vi "detect chassis.vi"(8 "error in":errorcluster, 11 "controller in":refnum<class "Controller.lvclass">) -> (0 "error out":errorcluster, 3 "controller out":refnum<class "Controller.lvclass">)   [LabVIEW 2014, in "SMI.lvlib" / "Controller.lvclass"]
uses:
  Controller.lvclass
  SysCfg Device/read system session.vi
  SysCfg Device/write system session.vi
  Chassis/Chassis.lvclass
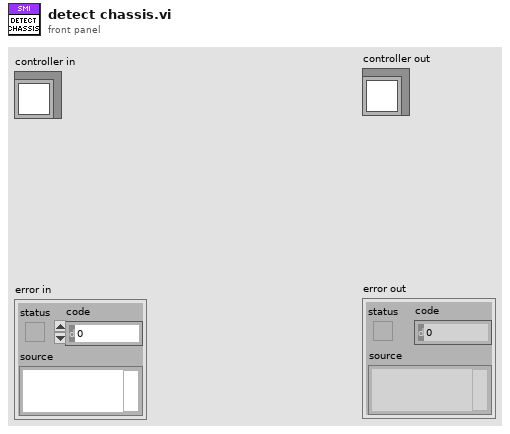
[diagram p1: front panel]
types:
  T1 = typedef "SMI.lvlib/Chassis.lvclass/chassis information.ctl" = cluster{"resource name":string, "vendor name":string, "product name":string, "product ID":u16, "serial number":string, "number of slots":i32, "device class":string}
  T2 = cluster{"local chassis":T1[], "remote chassis":T1[]}
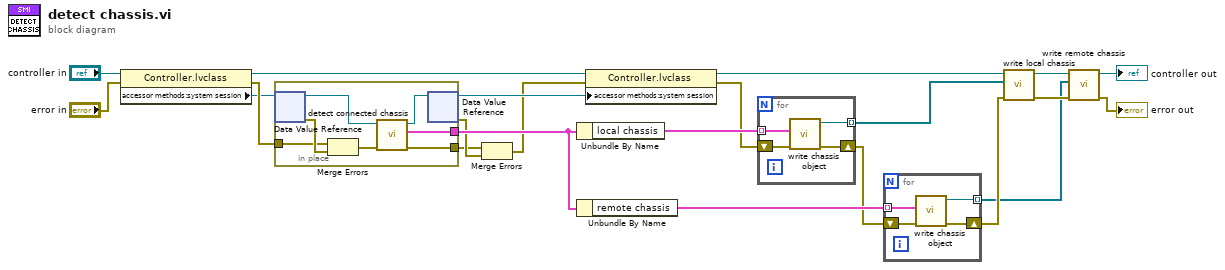
[diagram p0: block diagram]
diagram:
  n1 = property class="Controller.lvclass"(reference="controller in", error in="error in") -> (reference out=w20:refnum<class "Controller.lvclass">, error out=w22:errorcluster, "accessor methods:system session"=w5:refnum<data-value>)
  n2 = in-place {
    in-place-border: w22 -> [w24]
    in-place-border: [w29] -> w1
    in-place-border: [w28] -> w14
    n3 = in-place-dvr #1(w5) -> (w26:refnum<k21>, w25:errorcluster)
    n4 = Merge Errors(w24, w25) -> (w23:errorcluster)
    n5 = call "detect connected chassis.vi"("error in"=w23, "system session in"=w26) -> ("error out"=w29:errorcluster, "chassis"=w28:T2, "system session out"=w27:refnum<k21>)  [unwired: 7 in]
    n6 = in-place-dvr #1(w27) -> (w4:refnum<data-value>, w3:errorcluster)
  }
  n7 = Merge Errors(w1, w3) -> (w2:errorcluster)
  n8 = Unbundle By Name(w14) -> ("local chassis"=w12:T1[])
  n9 = Unbundle By Name(w14) -> ("remote chassis"=w13:T1[])
  n10 = property class="Controller.lvclass"(reference=w20, error in=w2, "accessor methods:system session"=w4) -> (reference out=w6:refnum<class "Controller.lvclass">, error out=w11:errorcluster)
  n11 = for {
    tunnel: w12 -> [w33] mode=indexing
    shift-right: [w31] -> w10
    shift-left: w11 -> [w32]
    tunnel: [w30] -> w9 mode=indexing
    n12 = call "write chassis object.vi"("error in"=w32, "chassis information"=w33) -> ("error out"=w31:errorcluster, "Chassis out"=w30:refnum<class "Chassis.lvclass">)  [unwired: 8 in]
  }
  n13 = for {
    tunnel: w13 -> [w37] mode=indexing
    shift-right: [w35] -> w15
    shift-left: w10 -> [w36]
    tunnel: [w34] -> w8 mode=indexing
    n14 = call "write chassis object.vi"("error in"=w36, "chassis information"=w37) -> ("error out"=w35:errorcluster, "Chassis out"=w34:refnum<class "Chassis.lvclass">)  [unwired: 8 in]
  }
  n15 = call "write local chassis.vi"("error in"=w15, "local chassis"=w9, "controller in"=w6) -> ("error out"=w16:errorcluster, "controller out"=w19:refnum<class "Controller.lvclass">)  [unwired: 7 in]
  n16 = call "write remote chassis.vi"("error in"=w16, "remote chassis"=w8, "controller in"=w19) -> ("error out"=→"error out":errorcluster, "controller out"=→"controller out":refnum<class "Controller.lvclass">)  [unwired: 7 in]
